vi "Replace Multiple Items at Offsets.vi"(8 "error in (no error)":errorcluster, 9 "New JSON Items":string[](array[string]), 10 "Offsets of Items to Replace":i32[](array[numeric]), 11 "JSON":string) -> (0 "error out":errorcluster, 3 "<JSON>":string)   [LabVIEW 2021, in "json.facade.lvlib"]
doc: "Replace the JSON Values located at Offsets in the input JSON. The Offsets can be that returned by a previous \"Find\" operation on the input JSON."
uses:
  json.facade.lvlib
  jsontext/JSONtext.lvlib
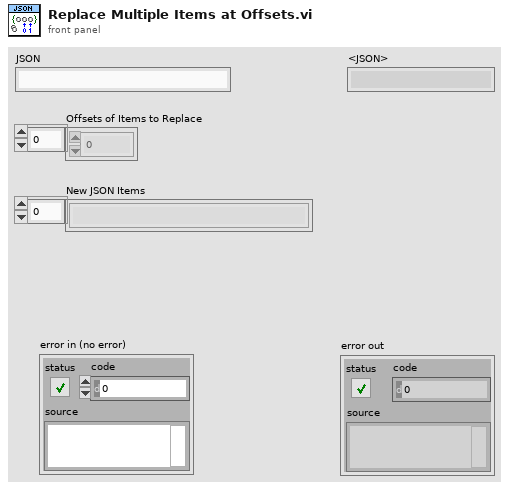
[diagram p1: front panel]
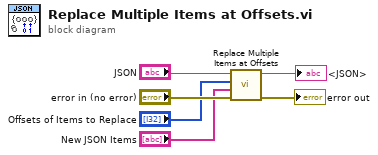
[diagram p0: block diagram]
diagram:
  n1 = call "Replace Multiple Items at Offsets.vi"("error in (no error)"="error in (no error)", "New JSON Items"="New JSON Items", "Offsets of Items to Replace"="Offsets of Items to Replace", "JSON"="JSON") -> ("error out"=→"error out":errorcluster, "<JSON>"=→"<JSON>":string)  [unwired: 6 in]
